vi "m1m3_getEvent_ForceActuatorSetpointWarning.vi"(8 "error in (no error)":errorcluster, 11 "logevent_ForceActuatorSetpointWarning_Ctl":T1) -> (0 "error out":errorcluster, 2 "function return":i32, 3 "logevent_ForceActuatorSetpointWarning_Ctl out":T1)   [LabVIEW 2016, in "SALLV_m1m3.lvlib"]
doc: "int m1m3_shm_getEvent_ForceActuatorSetpointWarningLV(m1m3_logevent_ForceActuatorSetpointWarningLV *logevent_ForceActuatorSetpointWarning_Ctl );"
uses:
  SALLV_m1m3.lvlib
  DataTypes/logevent_ForceActuatorSetpointWarning.ctl
  SALLV_m1m3.so
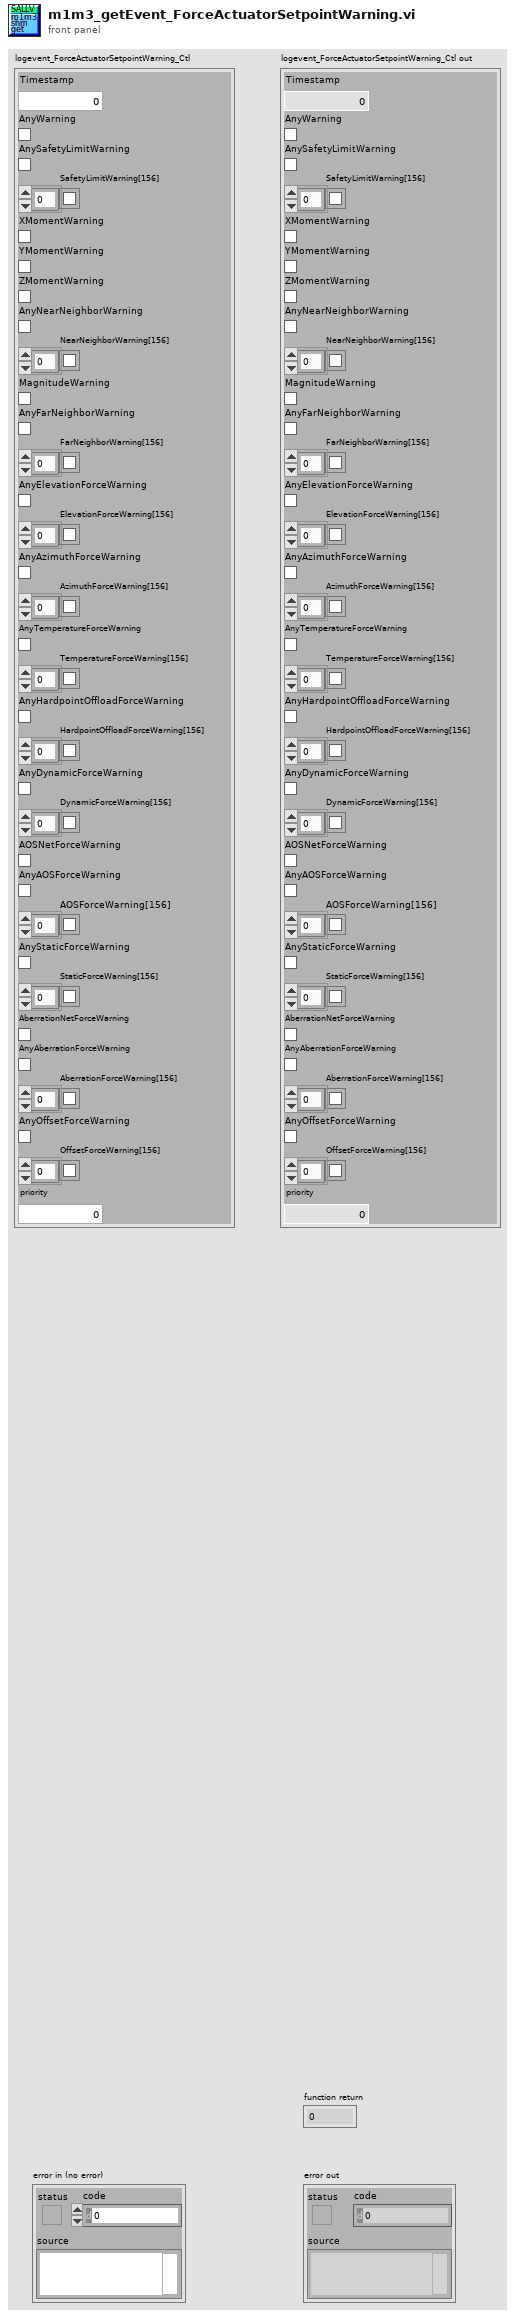
[diagram p1: front panel]
types:
  T1 = typedef "SALLV_m1m3.lvlib/logevent_ForceActuatorSetpointWarning.ctl" = cluster{"Timestamp":dbl, "AnyWarning":bool, "AnySafetyLimitWarning":bool, "SafetyLimitWarning[156]":bool[], "XMomentWarning":bool, "YMomentWarning":bool, "ZMomentWarning":bool, "AnyNearNeighborWarning":bool, "NearNeighborWarning[156]":bool[], "MagnitudeWarning":bool, "AnyFarNeighborWarning":bool, "FarNeighborWarning[156]":bool[], "AnyElevationForceWarning":bool, "ElevationForceWarning[156]":bool[], "AnyAzimuthForceWarning":bool, "AzimuthForceWarning[156]":bool[], "AnyTemperatureForceWarning":bool, "TemperatureForceWarning[156]":bool[], "AnyHardpointOffloadForceWarning":bool, "HardpointOffloadForceWarning[156]":bool[], "AnyDynamicForceWarning":bool, "DynamicForceWarning[156]":bool[], "AOSNetForceWarning":bool, "AnyAOSForceWarning":bool, "AOSForceWarning[156]":bool[], "AnyStaticForceWarning":bool, "StaticForceWarning[156]":bool[], "AberrationNetForceWarning":bool, "AnyAberrationForceWarning":bool, "AberrationForceWarning[156]":bool[], "AnyOffsetForceWarning":bool, "OffsetForceWarning[156]":bool[], "priority":i32}
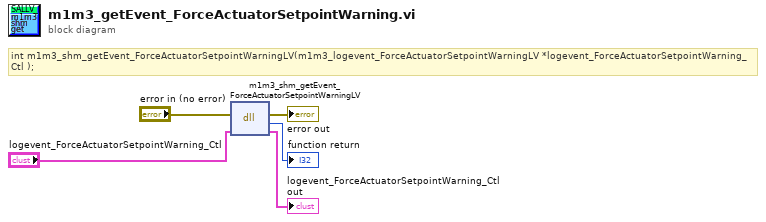
[diagram p0: block diagram]
diagram:
  # "int m1m3_shm_getEvent_ForceActuatorSetpointWarningLV(m1m3_logevent_ForceActuatorSetpointWarningLV *logevent_ForceActuatorSetpointWarning_Ctl );"
  n1 = dll-call lib="opt/CODE/SALLV_m1m3/SALLV_m1m3.*" fn="m1m3_shm_getEvent_ForceActuatorSetpointWarningLV"(error in="error in (no error)", "logevent_ForceActuatorSetpointWarning_Ctl"="logevent_ForceActuatorSetpointWarning_Ctl") -> (error out=→"error out":errorcluster, →"function return":i32, "logevent_ForceActuatorSetpointWarning_Ctl"=→"logevent_ForceActuatorSetpointWarning_Ctl out":T1)  [unwired: 2 in, 1 out]
